vi "Convert U8Cluster to U32 Representation.vi"(1 "U8 Cluster in":u8[](array[numeric])) -> (0 "U32 Cluster out":u32[](array[numeric]))   [LabVIEW 2018, in "FPGA Register IO.lvlib"]
uses:
  FPGA Register IO.lvlib
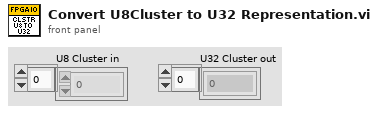
[diagram p1: front panel]
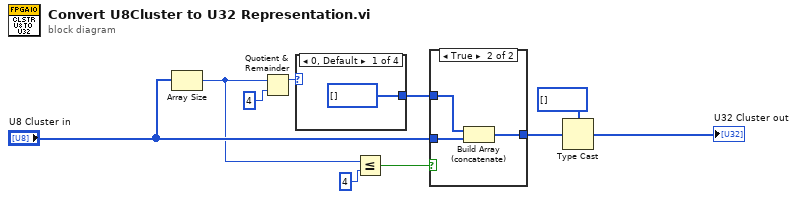
[diagram p0: block diagram]
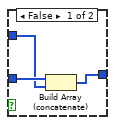
[diagram p2: hidden frame]
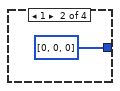
[diagram p3: hidden frame]
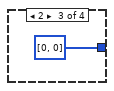
[diagram p4: hidden frame]
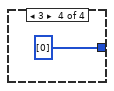
[diagram p5: hidden frame]
diagram:
  n1 = Array Size(array="U8 Cluster in") -> (size(s)=w6:i32)
  n2 = Quotient & Remainder(x=w6, y=4) -> (x-y*floor(x/y)=w4:i32)  [unwired: 1 out]
  n3 = case shown="0, Default" w4 {
    tunnel: [u8[] [] ("element") u8[] [0, 0, 0] ("element") u8[] [0, 0] ("element") u8[] [0] ("element")] -> w9
    frame 0, Default {
    }
    frame 1 {
    }
    frame 2 {
    }
    frame 3 {
    }
  }
  n4 = Less Or Equal?(x=w6, y=4) -> (x <= y?=w7:bool)
  n5 = case shown="True" w7 {
    tunnel: "U8 Cluster in" -> [w17 w19]
    tunnel: w9 -> [w16 w20]
    tunnel: [w15 w18] -> w10
    frame False {
      n6 = Build Array (concatenate)(w17, w16) -> (w15:u8[])
    }
    frame True {
      n7 = Build Array (concatenate)(w20, w19) -> (w18:u8[])
    }
  }
  n8 = Type Cast(type=u32[] [] ("bparray"), x=w10) -> (*(type *) &x=→"U32 Cluster out":u32[])
